vi "Get Application Name.vi"(8 "error in":errorcluster, 11 "Springboard Station Configuration in":refnum<class "Springboard Station Configuration.lvclass">) -> (0 "error out":errorcluster, 2 "Application Name":string, 3 "Springboard Station Configuration out":refnum<class "Springboard Station Configuration.lvclass">)   [LabVIEW 2018, in "Springboard TLB`.lvlib" / "Springboard Station Configuration.lvclass"]
uses:
  Springboard Station Configuration.lvclass
  Springboard Station Configuration.lvclass/Springboard Station Configuration.ctl
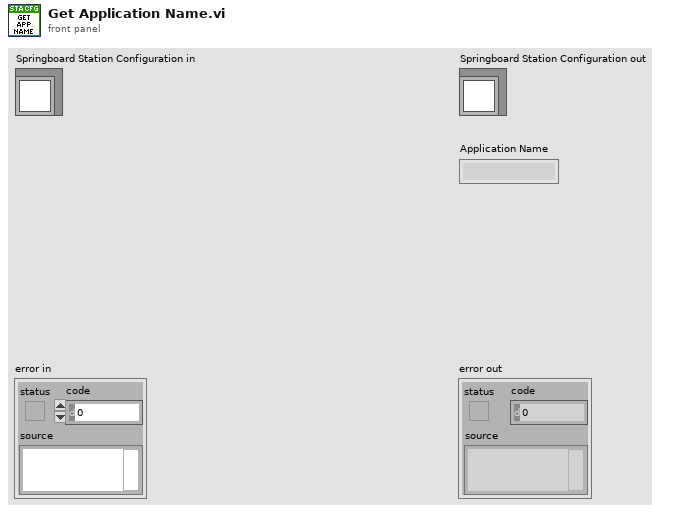
[diagram p1: front panel]
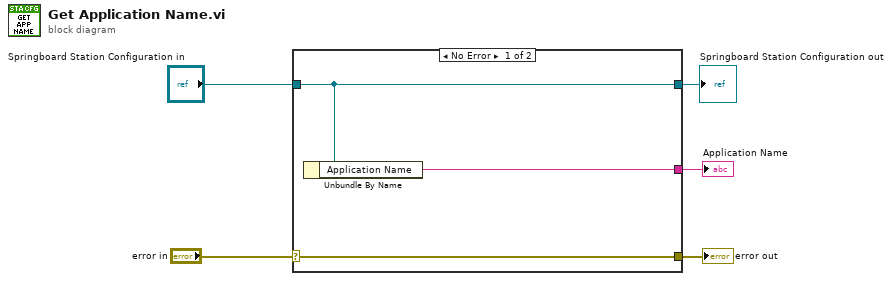
[diagram p0: block diagram]
diagram:
  n1 = case shown="No Error" "error in" {
    selector: "error in" -> [w8 w9]
    tunnel: [w8 w9] -> w4
    tunnel: [w7 w10] -> w2
    tunnel: "Springboard Station Configuration in" -> [w7 w10]
    tunnel: [w6 _] -> w1
    frame No Error {
      n2 = Unbundle By Name(w7) -> ("Application Name"=w6:string)
    }
    frame Error {
    }
  }
  "error out" <- w4
  "Springboard Station Configuration out" <- w2
  "Application Name" <- w1
